vi "Error Cluster from Fault.vi"(11 "Fault indicators":bool[](array[boolean])) -> (3 "error out":errorcluster)   [LabVIEW 2020, in "ChromTech Next Gen Pump.lvlib"]
uses:
  ChromTech Next Gen Pump.lvlib
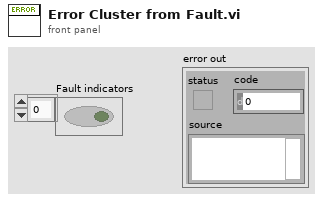
[diagram p1: front panel]
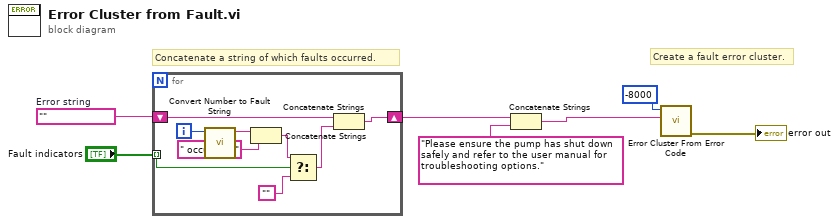
[diagram p0: block diagram]
diagram:
  w6 = ""  # Error string
  # "Create a fault error cluster."
  # "Concatenate a string of which faults occurred."
  n1 = for {
    tunnel: "Fault indicators" -> [w14] mode=indexing
    shift-right: [w15] -> w5
    shift-left: w6 -> [w16]
    i -> [w11]
    n2 = call "Convert Number to Fault String.vi"("Number"=w11) -> ("Fault String"=w10:string)  [unwired: 10 in]
    n3 = Concatenate Strings(w10, " occurred. " ("string")) -> (w9:string)
    n4 = Select(t=w9, s=w14, f="") -> (s? t:f=w13:string)
    n5 = Concatenate Strings(w16, w13) -> (w15:string)
  }
  n6 = Concatenate Strings(w5, "Please ensure the pump has shut down safely and refer to the user manual for troubleshooting options." ("string")) -> (w2:string)
  n7 = call <vilib>:"Error Cluster From Error Code.vi"("error message (\"\")"=w2, "error code (0)"=-8000) -> ("error out"=→"error out":errorcluster)  [unwired: 7 in]
